vi "ziExample-AUXIn.vi"() -> ()   [LabVIEW 2009]
doc: "Control a Zurich instrument device via the LabOne Labview API. \nRequirements: Zurich Instruments MFLI, HF2 or UHFLI \nThis vi controls the aux outputs and reads the aux inputs.\n\n© Zurich Instruments AG, www.zhinst.com"
uses:
  <vilib>/Utility/error.llb/DialogType.ctl
  <instrlib>/Zurich Instruments LabOne/Public/Utility/ziTicksToS_vector.vi
  <instrlib>/Zurich Instruments LabOne/Public/Data/ziGetEventAuxInSample.vi
  <instrlib>/Zurich Instruments LabOne/Zurich Instruments LabOne.lvlib
panel:
  out "Error Out":errorcluster
  in  "Address":string="DEV"
  out "Selected Device":string
  in  "ramp":bool caption="Ramp Aux Out"
  in  "Samples":u32=1000
  out "Progress":dbl(slide) scale=0.0..1.0
  in  "run":bool
  in  "stop":bool
  out "Waveform":cluster{"AuxInput":dbl[], "AuxInput":dbl[]}[](graph)
  # "Tested Instruments:\n- MFLI\n- HF2LI\n- UHFLI"
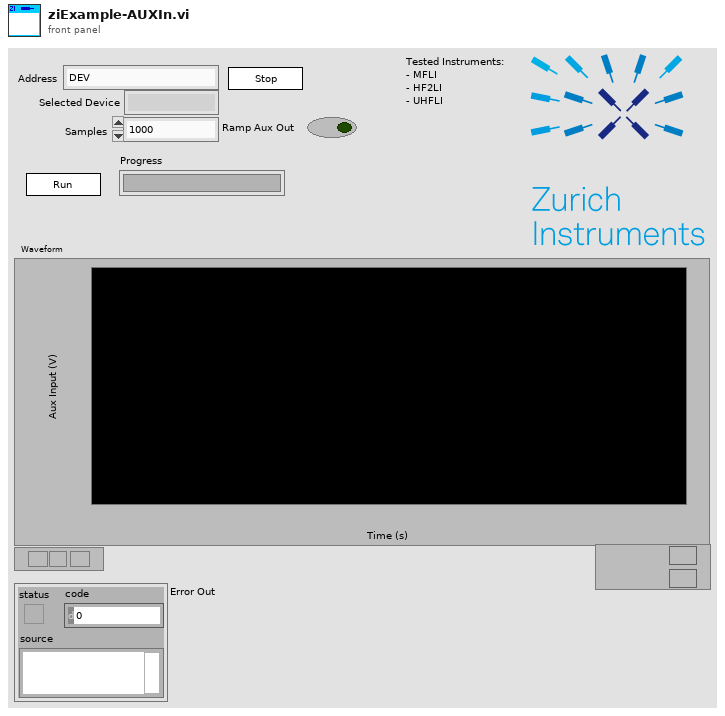
[diagram p1: front panel]
types:
  T1 = typedef "DialogType.ctl" = u16
  T2 = typedef "Zurich Instruments LabOne.lvlib/ziTypeHandle.ctl" = cluster{"handleValid":bool, "Conn":u64, "Path Prefix":string, "Handle":u64, "Connected":bool, "Clockbase(s)":dbl}
  T3 = typedef "Zurich Instruments LabOne.lvlib/ziTypePollType.ctl" = enum16{"NONE", "DOUBLE_DATA", "INTEGER_DATA", "DEMOD_SAMPLE", "SCOPE_WAVE_HF2", "AUXIN_SAMPLE", "DIO_SAMPLE", "BYTE_ARRAY", "PWA_WAVE", "9", "10", "11", "12", "13", "14", "15", "TREE_CHANGE_DEPRI", "17", "ERROR", "19", "20", "21", "22", "23", "24", "25", "26", "27", "28", "29", "30", "31", "DOUBLE_DATA_TS", "INTEGER_DATA_TS", "34", "SCOPE_WAVE", "36", "37", "BYTE_ARRAY_TS", "39", "40", "41", "42", "43", "44", "45", "CNT_DATA", "47", "TREE_CHANGE", "49", "50", "51", "52", "53", "54", "55", "56", "57", "58", "59", "60", "61", "62", "63", "SWEEPER_DATA", "SPECTRUM_DATA", "ADVISOR_DATA", "67", "IMP_DATA"}
  T4 = typedef "Zurich Instruments LabOne.lvlib/ziTypeAuxInSample.ctl" = cluster{"Timestamp (ticks)":u64[], "Val Ch0 (V)":dbl[], "Val Ch1 (V)":dbl[]}
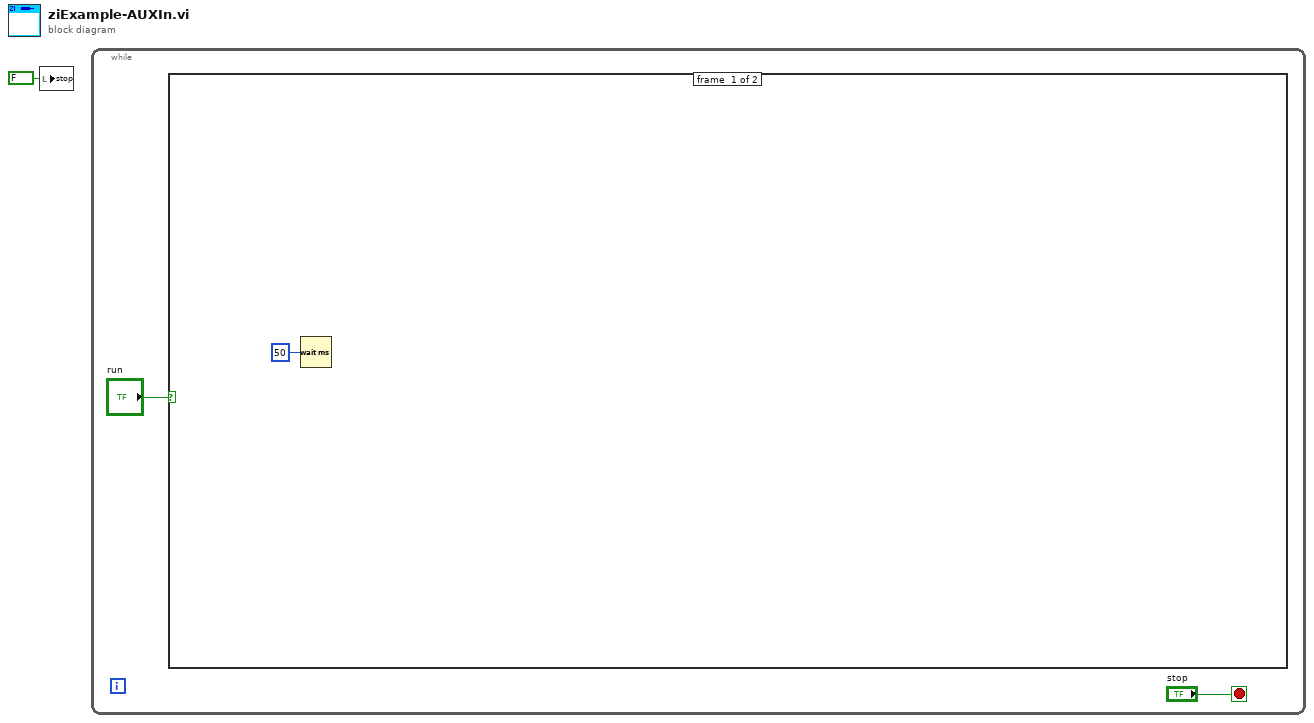
[diagram p0: block diagram]
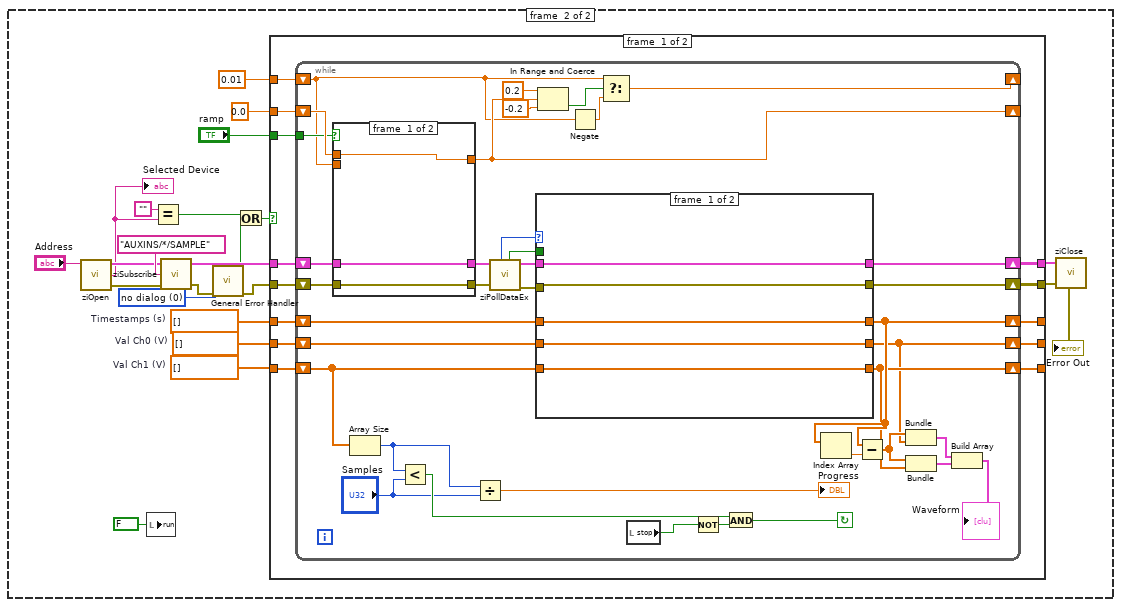
[diagram p2: hidden frame]
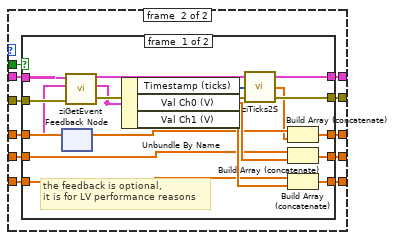
[diagram p3: hidden frame]
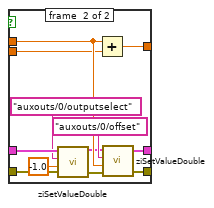
[diagram p5: hidden frame]
diagram:
  n1 = local write "stop"(FALSE ("run")) -> ()
  n2 = while {
    stop <- "stop" stop-if-true
    n3 = case shown="True" "run" {
      frame #0 {
        n4 = Wait (ms)(milliseconds to wait=50) -> ()  [unwired: 1 out]
      }
      frame #1 {
        w6 = T1 0 items=["no dialog", "OK message", "continue or stop message", "OK message + warnings", "continue/stop + warnings"] ("type of dialog (OK msg:1)")
        w21 = dbl[] []  # Val Ch1 (V)
        w22 = dbl[] []  # Val Ch0 (V)
        w23 = dbl[] []  # Timestamps (s)
        n5 = call <instrlib>:"ziOpen.vi"("Address"="Address") -> ("Error Out"=w14:errorcluster, "Selected Device"=w7:string, "HandleOut"=w13:T2)  [unwired: 1 in, 2 out]
        "Selected Device" <- w7
        n6 = local write "run"(FALSE ("run")) -> ()
        n7 = Equal?(x="", y=w7) -> (x = y?=w17:bool)
        n8 = call <instrlib>:"ziSubscribe.vi"("error in"=w14, "Path ()"="AUXINS/*/SAMPLE", "Handle In"=w13) -> ("error out"=w25:errorcluster, "Handle Out"=w27:T2)  [unwired: 1 out]
        n9 = call <vilib>:"General Error Handler.vi"("type of dialog (OK msg:1)"=w6, "error in (no error)"=w25) -> ("error?"=w19:bool, "error out"=w24:errorcluster)  [unwired: 9 in, 3 out]
        n10 = Or(x=w17, y=w19) -> (x .or. y?=w18:bool)
        n11 = case shown="False" w18 {
          tunnel: w27 -> [w40 w136]
          tunnel: [w39 w136] -> w16
          tunnel: [w38 w135] -> w15
          tunnel: [w37 w132] -> _
          tunnel: 0.0 -> [w36 _]
          tunnel: 0.01 -> [w35 _]
          tunnel: "ramp" -> [w34 _]
          tunnel: w24 -> [w33 w135]
          tunnel: w21 -> [w32 w132]
          tunnel: w23 -> [w31 w134]
          tunnel: w22 -> [w30 w133]
          tunnel: [w29 w134] -> _
          tunnel: [w28 w133] -> _
          frame #0 {
            n12 = while {
              shift-right: [w42] -> w37
              shift-left: w32 -> [w66]
              shift-right: [w61] -> w39
              shift-left: w40 -> [w74]
              shift-right: [w59] -> w38
              shift-left: w33 -> [w75]
              shift-right: [w51] -> _
              shift-left: w36 -> [w73]
              shift-right: [w70] -> _
              shift-left: w35 -> [w49]
              tunnel: w34 -> [w69]
              shift-right: [w43] -> w29
              shift-left: w31 -> [w65]
              shift-right: [w41] -> w28
              shift-left: w30 -> [w64]
              stop <- w58 continue-if-true
              n13 = case shown="True" w69 {
                tunnel: w75 -> [w118 w125]
                tunnel: w74 -> [w117 w126]
                tunnel: w73 -> [w119 w130]
                tunnel: w49 -> [_ w120]
                tunnel: [w119 w129] -> w51
                tunnel: [w118 w128] -> w72
                tunnel: [w117 w127] -> w71
                frame #0 {
                }
                frame #1 {
                  n14 = call <instrlib>:"ziSetValueDouble.vi"("Error In"=w125, "Value"=-1.0, "Path"="auxouts/0/outputselect", "Handle In"=w126) -> ("Error Out"=w124:errorcluster, "Handle Out"=w123:T2)  [unwired: 1 out]
                  n15 = Add(x=w130, y=w120) -> (x+y=w129:dbl)
                  n16 = call <instrlib>:"ziSetValueDouble.vi"("Error In"=w124, "Value"=w130, "Path"="auxouts/0/offset", "Handle In"=w123) -> ("Error Out"=w128:errorcluster, "Handle Out"=w127:T2)  [unwired: 1 out]
                }
              }
              n17 = Array Size(array=w66) -> (size(s)=w67:i32)
              n18 = Less?(x=w67, y="Samples") -> (x < y?=w76:bool)
              n19 = Divide(x=w67, y="Samples") -> (x/y=→"Progress":dbl)
              n20 = call <instrlib>:"ziPollDataEx.vi"("error in"=w72, "Handle In"=w71) -> ("error out"=w60:errorcluster, "Handle Out"=w62:T2, "Timed Out"=w77:bool, "ziValueType"=w55:T3)  [unwired: 2 in, 4 out]
              n21 = case shown="\"AUXIN_SAMPLE\"" w55 {
                tunnel: w77 -> [_ w93]
                tunnel: w66 -> [w78 w92]
                tunnel: w65 -> [w80 w91]
                tunnel: w64 -> [w79 w90]
                tunnel: [w78 w89] -> w42
                tunnel: [w80 w88] -> w43
                tunnel: [w79 w87] -> w41
                tunnel: w62 -> [w82 w86]
                tunnel: [w82 w85] -> w61
                tunnel: w60 -> [w81 w84]
                tunnel: [w81 w83] -> w59
                frame #0 {
                }
                frame #1 {
                  n22 = case shown="False" w93 {
                    tunnel: w92 -> [w107 w114]
                    tunnel: w91 -> [w109 w116]
                    tunnel: w90 -> [w108 w115]
                    tunnel: [w106 w114] -> w89
                    tunnel: [w105 w116] -> w88
                    tunnel: [w104 w115] -> w87
                    tunnel: w86 -> [w103 w113]
                    tunnel: [w101 w113] -> w85
                    tunnel: w84 -> [w102 w112]
                    tunnel: [w97 w112] -> w83
                    frame #0 {
                      # "the feedback is optional, \nit is for LV performance reasons"
                      n23 = feedback #1() -> (w95:T4)  [unwired: 1 in]
                      n24 = call-poly <instrlib>:"ziGetEvent.vi"("Error In"=w102, "AuxIn In"=w95, "Handle In"=w103) -> ("Error Out"=w98:errorcluster, "AuxIn Out"=w94:T4, "Handle Out"=w99:T2)  [unwired: 6 in]
                      n25 = Unbundle By Name(w94) -> ("Timestamp (ticks)"=w100:u64[], "Val Ch0 (V)"=w111:dbl[], "Val Ch1 (V)"=w110:dbl[])
                      n26 = call-poly <instrlib>:"ziTicks2S.vi"("Error In"=w98, "Timestamp (ticks)"=w100, "Handle In"=w99) -> ("Error Out"=w97:errorcluster, "Timestamp(s)"=w96:dbl[], "Handle Out"=w101:T2)
                      n27 = Build Array (concatenate)(w109, w96) -> (w105:dbl[])
                      n28 = Build Array (concatenate)(w108, w111) -> (w104:dbl[])
                      n29 = Build Array (concatenate)(w107, w110) -> (w106:dbl[])
                    }
                    frame #1 {
                    }
                  }
                }
              }
              n30 = In Range and Coerce(upper limit=0.2 ("y"), x=w51, lower limit=-0.2 ("y")) -> (In Range?=w52:bool)  [unwired: 1 out]
              n31 = Negate(x=w49) -> (-x=w50:dbl)
              n32 = Select(t=w49, s=w52, f=w50) -> (s? t:f=w70:dbl)
              n33 = local read "stop"() -> (w57:bool)
              n34 = Not(x=w57) -> (.not. x?=w56:bool)
              n35 = And(x=w76, y=w56) -> (x .and. y?=w58:bool)
              n36 = Index Array(array=w43) -> (element=w47:dbl)  [unwired: 1 in]
              n37 = Subtract(x=w43, y=w47) -> (x-y=w48:dbl[])
              n38 = Bundle(w48, "Val Ch0 (V)"=w41) -> (w44:cluster{dbl[], "Val Ch0 (V)":dbl[]})  [unwired: 1 out]
              n39 = Bundle(w48, "Val Ch1 (V)"=w42) -> (w45:cluster{dbl[], "Val Ch1 (V)":dbl[]})  [unwired: 1 out]
              n40 = Build Array(w44, w45) -> (→"Waveform":cluster{dbl[], "Val Ch1 (V)":dbl[]}[])
            }
          }
          frame #1 {
          }
        }
        n41 = call <instrlib>:"ziClose.vi"("Error In"=w15, "Handle In"=w16) -> ("Error Out"=→"Error Out":errorcluster)  [unwired: 3 out]
      }
    }
  }
